vi "PI_Picture_dyn_scanner_prepare.vi"(8 "Input Cluster":T6) -> (2 "Measurement time / [s]":u32, 3 "Commandset out":string[](array[string]))   [LabVIEW 2009]
uses:
  atmcd32d.llb/AcquisitionMode_mode typedef.ctl
  atmcd32d.llb/ReadMode_mode typedef.ctl
  atmcd32d.llb/TriggerMode_mode typedef.ctl
  atmcd32d.llb/Shutter_type typedef.ctl
  atmcd32d.llb/Shutter_mode typedef.ctl
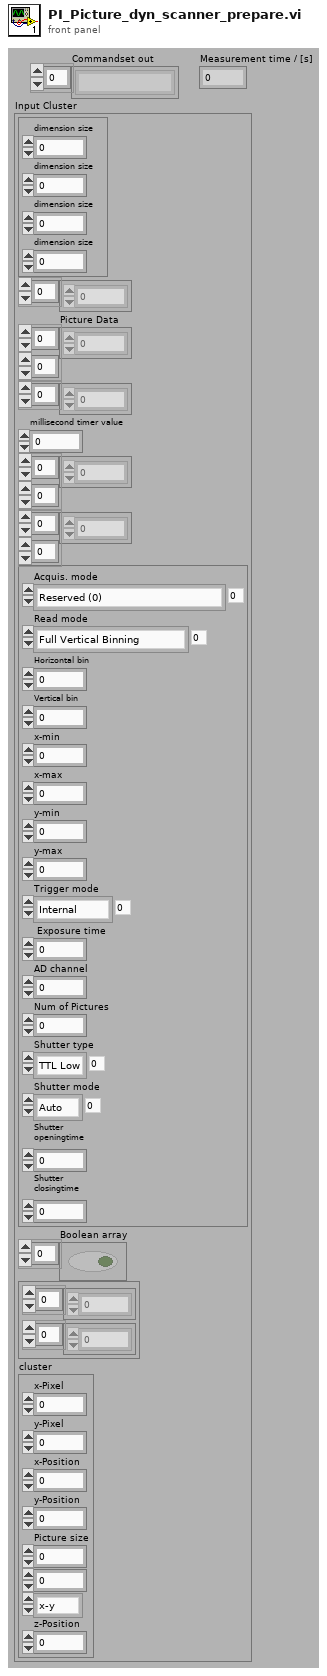
[diagram p1: front panel]
types:
  T1 = typedef "AcquisitionMode_mode typedef.ctl" = enum16{"Reserved (0)", "Single Scan", "Accumulate", "Kinetics", "Fast Kinetics", "Run Till Abort", "Reserved (6)", "Reserved (7)", "Reserved (8)", "Time Delayed Integration"}
  T2 = typedef "ReadMode_mode typedef.ctl" = enum16{"Full Vertical Binning", "Multi-Track", "Random-Track", "Single-Track", "Image"}
  T3 = typedef "TriggerMode_mode typedef.ctl" = enum16{"Internal", "External", "N/A (2)", "N/A (3)", "N/A (4)", "N/A (5)", "External Start"}
  T4 = typedef "Shutter_type typedef.ctl" = enum16{"TTL Low", "TTL High"}
  T5 = typedef "Shutter_mode typedef.ctl" = enum16{"Auto", "Open", "Close"}
  T6 = cluster{cluster{"dimension size":i32, "dimension size":i32, "dimension size":i32, "dimension size":i32}, i32[], "Picture Data":dbl[][], u32[], "millisecond timer value":u32, dbl[][], i32[][], cluster{"Acquis. mode":T1, "Read mode":T2, "Horizontal bin":i32, "Vertical bin":i32, "x-min":i32, "x-max":i32, "y-min":i32, "y-max":i32, "Trigger mode":T3, " Exposure time":sgl, "AD channel":i32, "Num of Pictures":i32, "Shutter type":T4, "Shutter mode":T5, "Shutter\nopeningtime":i32, "Shutter\nclosingtime":i32}, "Boolean array":bool[], cluster{dbl[], dbl[]}, "cluster":cluster{"x-Pixel":u16, "y-Pixel":u16, "x-Position":dbl, "y-Position":dbl, "Picture size":dbl, dbl, enum32{"x-y", "x-z", "y-z"}, "z-Position":dbl}}
  T7 = cluster{"x-Pixel":u16, "y-Pixel":u16, "x-Position":dbl, "y-Position":dbl, "Picture size":dbl, dbl, enum32{"x-y", "x-z", "y-z"}, "z-Position":dbl}
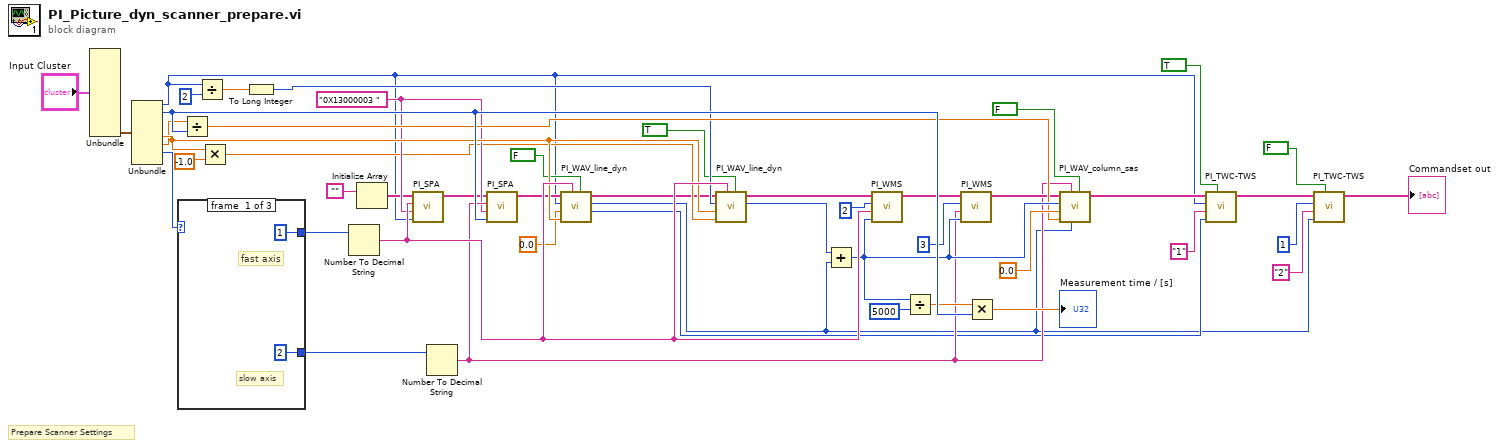
[diagram p0: block diagram]
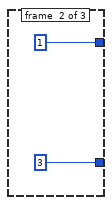
[diagram p2: hidden frame]
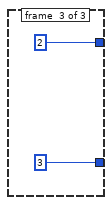
[diagram p3: hidden frame]
diagram:
  w30 = "0X13000003 " ("string")
  # "Prepare Scanner Settings"
  n1 = Unbundle("Input Cluster") -> ("cluster"=w1:T7)  [unwired: 10 out]
  n2 = Unbundle(w1) -> ("x-Pixel"=w10:u16, "y-Pixel"=w47:u16, "Picture size"=w42:dbl, w35:dbl, w15:enum32{"x-y", "x-z", "y-z"})  [unwired: 3 out]
  n3 = case shown="\"x-y\", Default" w15 {
    tunnel: [1 1 2] -> w16
    tunnel: [2 3 3] -> w17
    frame #0 {
      # "slow axis"
      # "fast axis"
    }
    frame #1 {
    }
    frame #2 {
    }
  }
  n4 = Divide(x=w35, y=w47) -> (x/y=w39:dbl)
  n5 = Divide(x=w10, y=u16 2) -> (x/y=w22:dbl)
  n6 = Multiply(x=w42, y=-1.0) -> (x*y=w24:dbl)
  n7 = To Long Integer(number=w22) -> (32bit integer=w23:i32)
  n8 = Number To Decimal String(number=w16) -> (decimal integer string=w48:string)  [unwired: 1 out]
  n9 = Initialize Array("") -> (w28:string[])  [unwired: 1 out]
  n10 = call "PI_SPA.vi"("Value"=w10, "Register"=w30, "Axis"=w48, "Commandset in"=w28) -> ("Commandset out"=w29:string[])  [unwired: 7 out]
  n11 = Number To Decimal String(number=w17) -> (decimal integer string=w37:string)  [unwired: 1 out]
  n12 = call "PI_SPA.vi"("Value"=w47, "Register"=w30, "Axis"=w37, "Commandset in"=w29) -> ("Commandset out"=w27:string[])  [unwired: 7 out]
  n13 = call "PI_WAV_line_dyn.vi"("Attach to wav"=FALSE, "Axis Identifier"=w48, "Amplitude / [mu]"=w42, "Startpos / [mu]"=0.0, "Pixel per scan"=w10, "Commandset in"=w27) -> ("Curve-Start-Pixel"=w12:i32, "Num_Pix"=w3:u16, "Commandset out"=w19:string[])  [unwired: 3 out]
  n14 = call "PI_WAV_line_dyn.vi"("Attach to wav"=TRUE, "Axis Identifier"=w48, "Amplitude / [mu]"=w24, "Startpos / [mu]"=w42, "Pixel per scan"=w23, "Commandset in"=w19) -> ("Num_Pix"=w26:u16, "Commandset out"=w31:string[])  [unwired: 4 out]
  n15 = Add(x=w26, y=w3) -> (x+y=w43:u16)
  n16 = call "PI_WMS.vi"("Pixels to reserve"=w43, "Axis"=w48, "Position / Commandset"=2, "Commandset in"=w31) -> ("Commandset out"=w32:string[])  [unwired: 7 out]
  n17 = Divide(x=w43, y=u16 5000) -> (x/y=w45:dbl)
  n18 = call "PI_WMS.vi"("Pixels to reserve"=w43, "Axis"=w37, "Position / Commandset"=3, "Commandset in"=w32) -> ("Commandset out"=w38:string[])  [unwired: 7 out]
  n19 = Multiply(x=w45, y=w47) -> (x*y=→"Measurement time / [s]":dbl)
  n20 = call "PI_WAV_column_sas.vi"("Attach to wav"=FALSE, "Steps per Scan-line"=w3, "Axis Identifier"=w37, "Amplitude / [mu]"=w39, "Startpos / [mu]"=0.0, "Pixel per scan"=w43, "Commandset in"=w38) -> ("Commandset out"=w13:string[])  [unwired: 4 out]
  n21 = call "PI_TWC-TWS.vi"("TWC?"=TRUE, "Curve_Start_Pixel"=w12, "Axis Identifier"="1", "Pixel per scan"=w10, "Commandset in"=w13) -> ("Commandset out"=w8:string[])  [unwired: 6 out]
  n22 = call "PI_TWC-TWS.vi"("TWC?"=FALSE, "Curve_Start_Pixel"=w3, "Axis Identifier"="2", "Pixel per scan"=u16 1, "Commandset in"=w8) -> ("Commandset out"=→"Commandset out":string[])  [unwired: 6 out]
